vi "WriteSetSize.vi"(8 "error in (no error)":errorcluster, 10 "Size":cluster{"Width":i16, "Height":i16}, 11 "reference in":refnum<class "Pgui_Obj.lvclass">) -> (0 "error out":errorcluster, 3 "reference out":refnum<class "Pgui_Obj.lvclass">)   [LabVIEW 2019, in "Pgui_Obj.lvclass"]
doc: "Sets Width And height of object"
uses:
  Pgui_Obj.lvclass
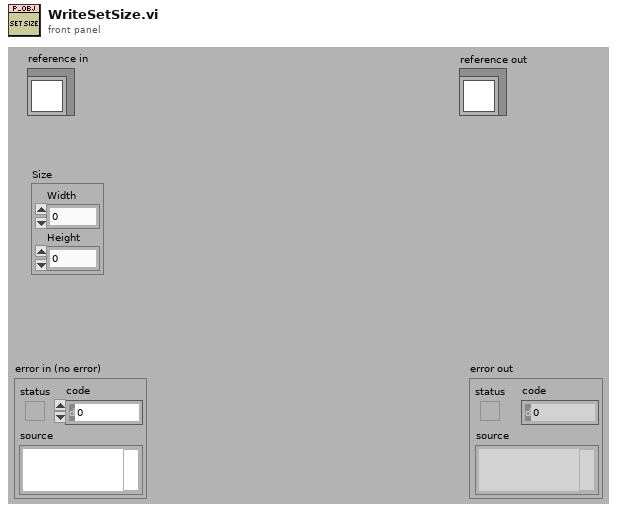
[diagram p1: front panel]
types:
  T1 = typedef "Pgui_Obj.lvclass/ObjectAttributes.ctl" = cluster{"Children":refnum<class "Pgui_Obj.lvclass">[], "Draw Instr":picture, "Params":cluster{"left":i16, "top":i16, "right":i16, "bottom":i16}, "Parent_Pgui_Obj":refnum<class "Pgui_Obj.lvclass">, "MouseOver":bool}
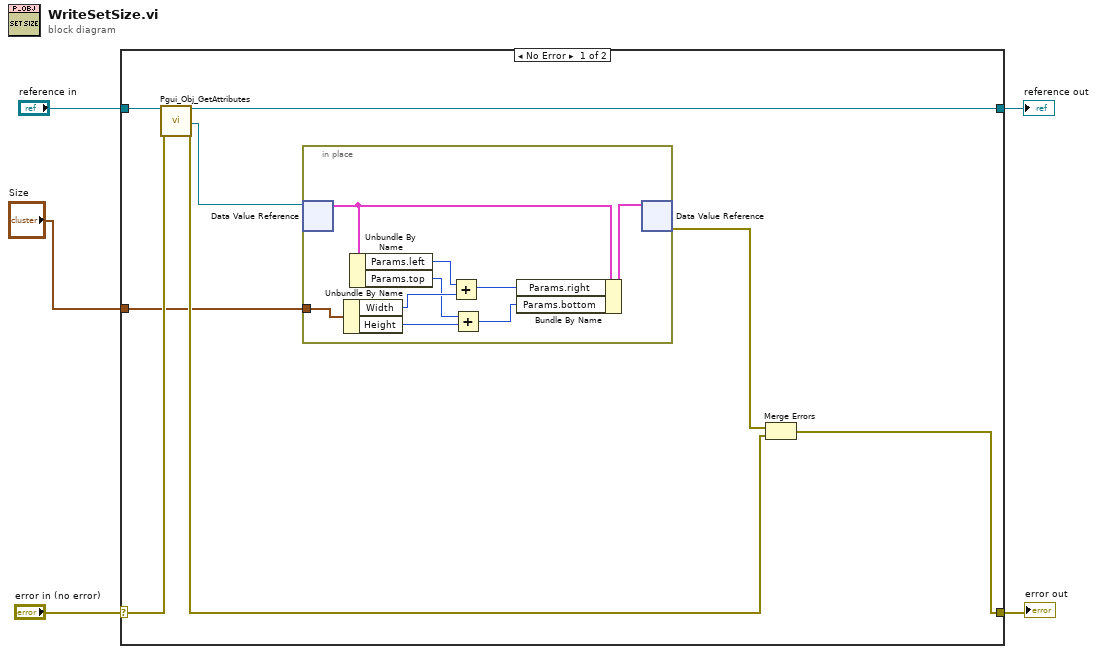
[diagram p0: block diagram]
diagram:
  n1 = case shown="No Error" "error in (no error)" {
    selector: "error in (no error)" -> [w13 w24]
    tunnel: [w8 w24] -> w4
    tunnel: [w11 w23] -> w2
    tunnel: "reference in" -> [w12 w23]
    tunnel: "Size" -> [w6 _]
    frame No Error {
      n2 = call "Pgui_Obj_GetAttributes.vi"("reference in"=w12, "error in (no error)"=w13) -> ("reference out"=w11:refnum<class "Pgui_Obj.lvclass">, "DataRef"=w7:refnum<data-value>, "error out"=w9:errorcluster)  [unwired: 14 in, 1 out]
      n3 = in-place {
        in-place-border: w6 -> [w19]
        n4 = in-place-dvr #1(w7) -> (w21:T1)  [unwired: 1 out]
        n5 = Unbundle By Name(w19) -> ("Width"=w18:i16, "Height"=w15:i16)
        n6 = Unbundle By Name(w21) -> ("Params.left"=w20:i16, "Params.top"=w16:i16)
        n7 = Add(x=w20, y=w18) -> (x+y=w17:i16)
        n8 = Add(x=w16, y=w15) -> (x+y=w14:i16)
        n9 = Bundle By Name(cluster=w21, "Params.right"=w17, "Params.bottom"=w14) -> (w22:T1)
        n10 = in-place-dvr #1(w22) -> (w10:errorcluster)  [unwired: 1 out]
      }
      n11 = Merge Errors(w10, w9) -> (w8:errorcluster)
    }
    frame Error {
    }
  }
  "error out" <- w4
  "reference out" <- w2
